vi "Esercitazione 3 - Struttura IF innestati.vi"() -> ()   [LabVIEW 2018]
panel:
  out "S1 == S2":bool
  out "S1 < S2":bool
  out "S1 > S2":bool
  in  "S2":string
  in  "S1":string
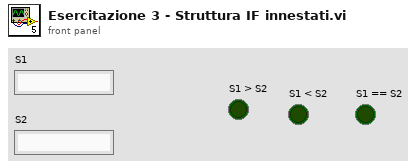
[diagram p1: front panel]
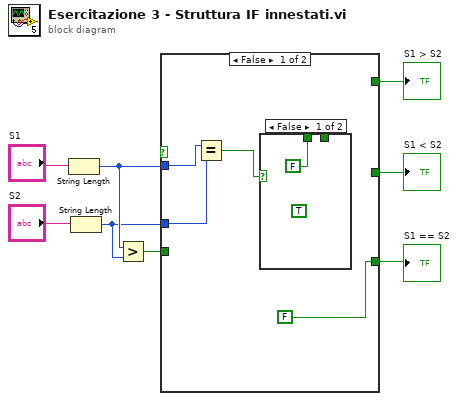
[diagram p0: block diagram]
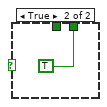
[diagram p2: hidden frame]
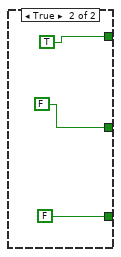
[diagram p3: hidden frame]
diagram:
  n1 = String Length(string="S1") -> (length=w6:i32)
  n2 = String Length(string="S2") -> (length=w5:i32)
  n3 = Greater?(x=w6, y=w5) -> (0:w4:bool)
  n4 = case shown="False" {
    selector: _ -> [_ _]
    tunnel: w6 -> [w11 _]
    tunnel: w5 -> [w10 _]
    tunnel: w4 -> [_ _]
    tunnel: [_ TRUE] -> w3
    tunnel: [_ FALSE] -> w2
    tunnel: [FALSE FALSE] -> w1
    frame False {
      n5 = Equal?(x=w11, y=w10) -> (x = y?=w12:bool)
      n6 = case shown="False" w12 {
        tunnel: [FALSE _] -> _
        tunnel: [_ TRUE] -> _
        frame False {
          (unwired) TRUE
        }
        frame True {
        }
      }
    }
    frame True {
    }
  }
  "S1 > S2" <- w3
  "S1 < S2" <- w2
  "S1 == S2" <- w1
